vi "Notifications-Events OverSampling x86.vi"() -> ()   [LabVIEW 2020]
uses:
  <userlib>/Beckhoff-LabVIEW-Interface/Utilities/Notification/Buffered User-Event Data.ctl
  <userlib>/Beckhoff-LabVIEW-Interface/_DependsOn/Base/Read/Register E-Notification Buffered.vi
panel:
  out "# elements in queue":i32
  out "Timestamps":i64[](graph)
  out "Signal":dbl[](graph)
  out "Has stopped?":bool
  in  "Stop Event-Loop":bool
  in  "Stop Notification":bool
  in  "Send":bool=TRUE
  in  "Symbol file path":path
  # "Stop Notification before stopping\nEvent-loop"
  # "Note: This example is only an illustration of all possible ways\nhow this Product can be used."
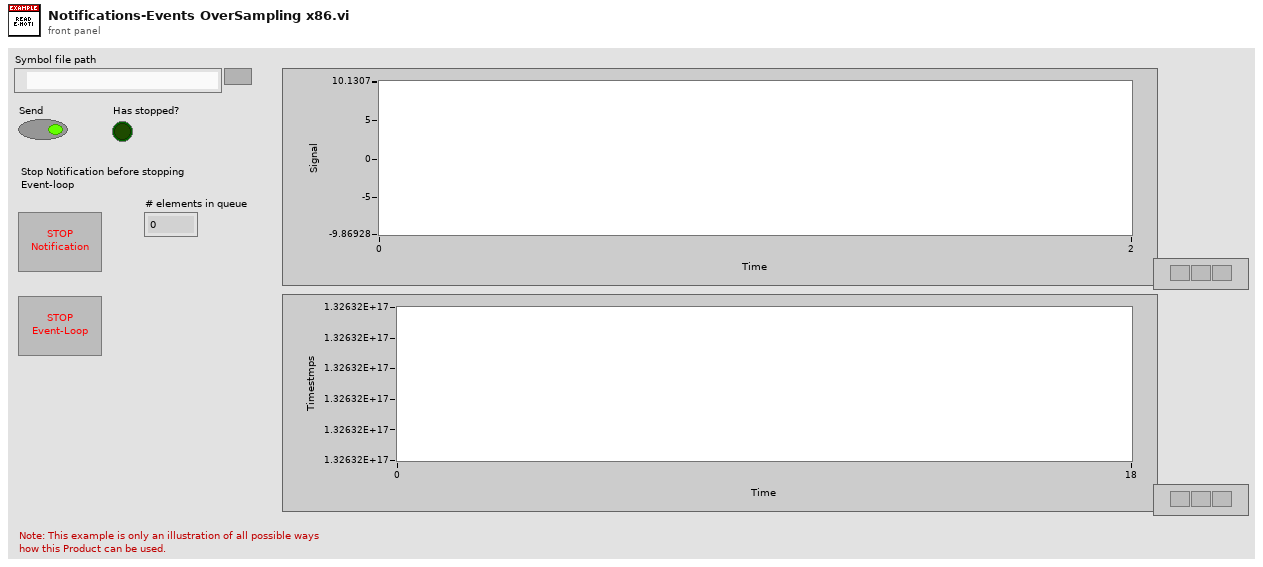
[diagram p1: front panel]
types:
  T1 = typedef "Buffered User-Event Data.ctl" = cluster{"NotiHandle":u32, "Samples":i32, "BufferInfo":cluster{"Previous Overflow Samples":u32, "Missing Samples":u32, "Buffer Usage":dbl}, "RawData":u8[], "Timestamps":i64[]}
  T2 = cluster{"Noti. Data":variant[], "Timestamps":i64[]}
  T3 = cluster{"RDataArray":variant[], "Timestamps":i64[]}
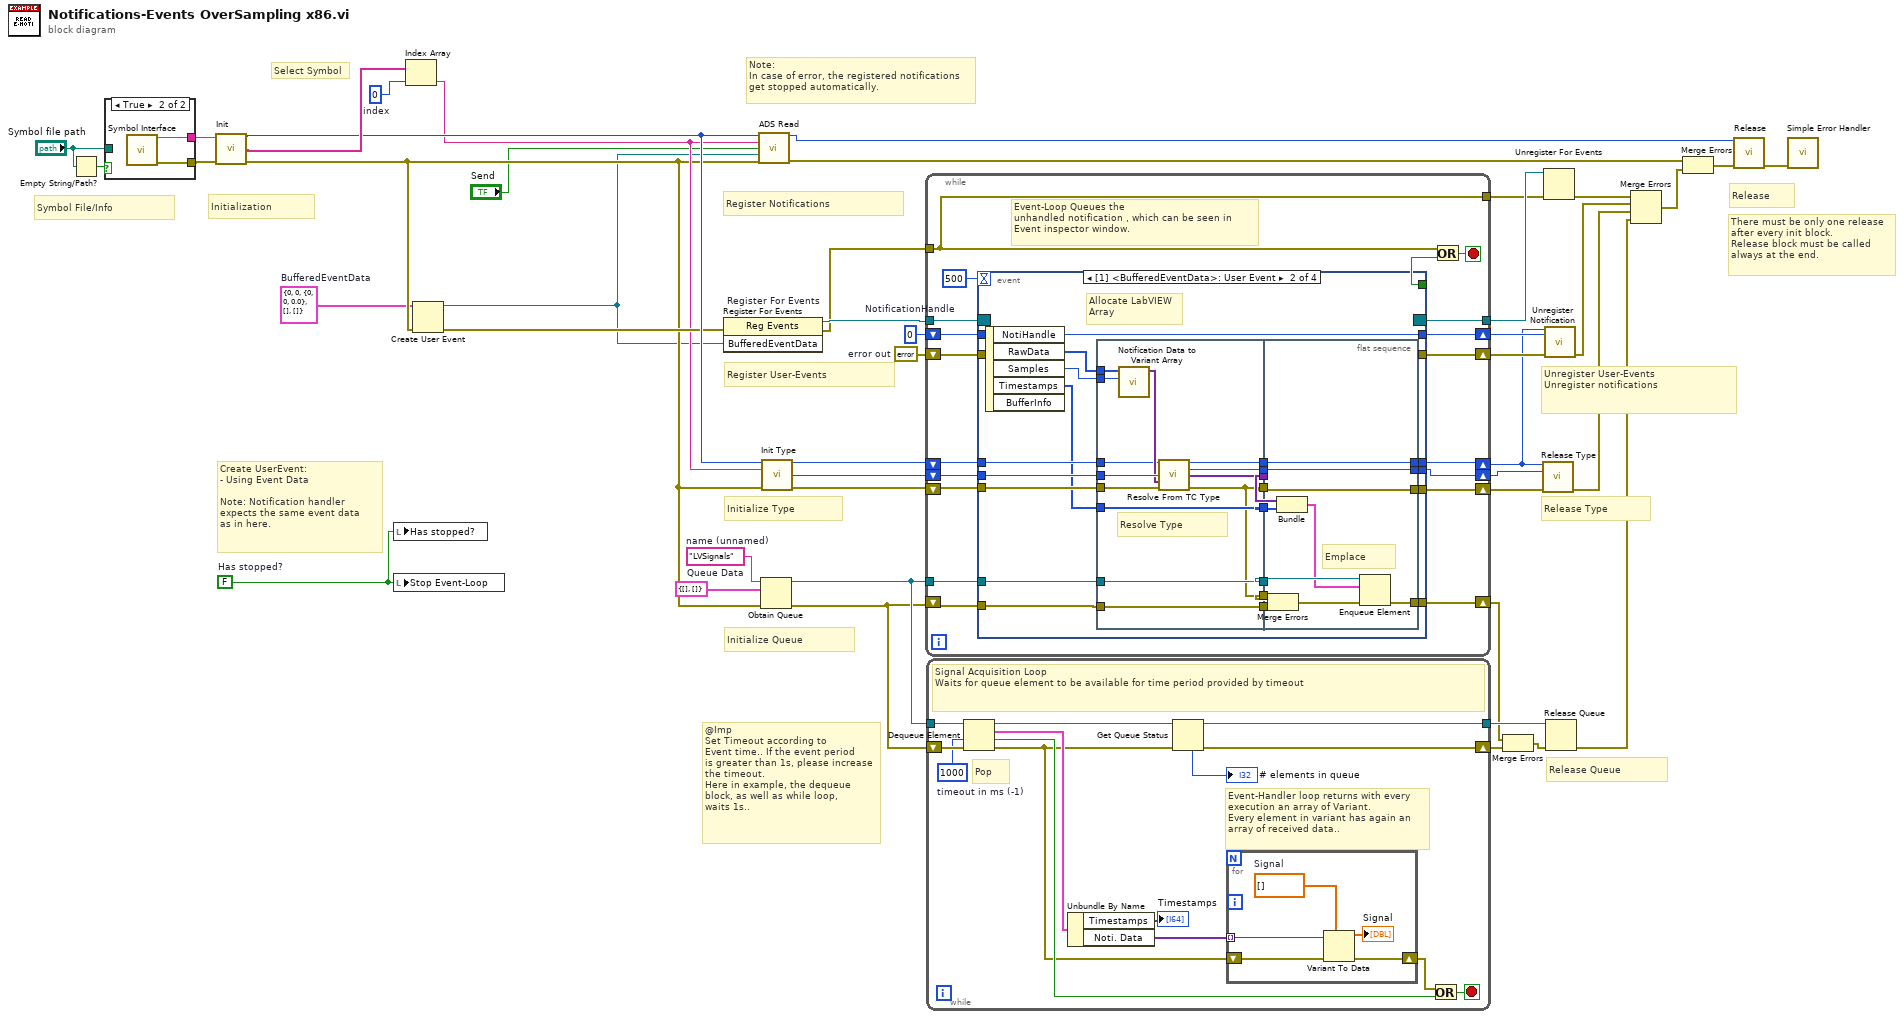
[diagram p0: block diagram]
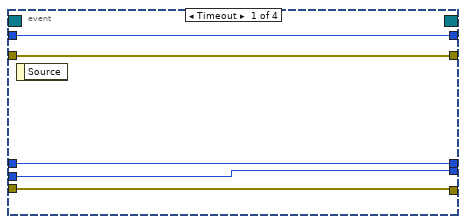
[diagram p2: hidden frame]
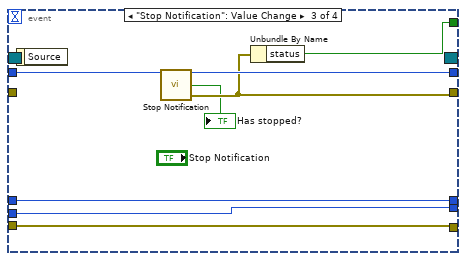
[diagram p3: hidden frame]
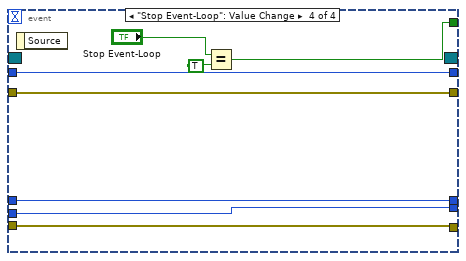
[diagram p4: hidden frame]
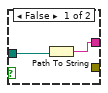
[diagram p5: hidden frame]
diagram:
  w3 = T1 {"NotiHandle"=0, "Samples"=0, "BufferInfo"={"Previous Overflow Samples"=0, "Missing Samples"=0, "Buffer Usage"=0.0}, "RawData"=[], "Timestamps"=[]}  # BufferedEventData
  w13 = "LVSignals"  # name (unnamed)
  w14 = T2 {"Noti. Data"=[], "Timestamps"=[]}  # Queue Data
  w23 = errorcluster {"status"=FALSE, "code"=0, "source"=""}  # error out
  w24 = u32 0  # NotificationHandle
  w36 = 0  # index
  w6 = FALSE  # Has stopped?
  # "@Imp\nSet Timeout according to\nEvent time.. If the event period\nis greater than 1s, please increase\nthe timeout.\nHere in example, the dequeue\nblock, as well as while loop,\nwaits 1s.."
  # "Release Queue"
  # "Initialize Queue"
  # "Release Type"
  # "Initialize Type"
  # "Note:\nIn case of error, the registered notifications\nget stopped automatically."
  # "There must be only one release\nafter every init block.\nRelease block must be called\nalways at the end."
  # "Create UserEvent:\n- Using Event Data\n\nNote: Notification handler\nexpects the same event data\nas in here."
  # "Unregister User-Events\nUnregister notifications"
  # "Register User-Events"
  # "Register Notifications"
  # "Initialization"
  # "Select Symbol"
  # "Release"
  # "Symbol File/Info"
  n1 = Empty String/Path?(string/path="Symbol file path") -> (empty?=w40:bool)
  n2 = case shown="True" w40 {
    tunnel: [_ w49] -> w39
    tunnel: [w47 w48] -> w38
    tunnel: "Symbol file path" -> [w46 _]
    frame False {
      n3 = Path To String(path=w46) -> (string=w47:string)
    }
    frame True {
      n4 = call <userlib>:"Symbol Interface.vi"() -> ("PortInfo"=w48:string, "error out"=w49:errorcluster)  [unwired: 14 in]
    }
  }
  n5 = call <userlib>:"Init.vi"("XMLDescription"=w38, "error in (no error)"=w39) -> ("Handle"=w41:u32, "ReadGrpSymbols"=w45:string[], "error out"=w12:errorcluster)  [unwired: 9 in, 2 out]
  n6 = local write "Has stopped?"(w6) -> ()
  n7 = local write "Stop Event-Loop"(w6) -> ()
  n8 = Index Array "Index Array"(array=w45, index=w36) -> (element=w22:string)
  n9 = Create User Event(user event datatype=w3, error in=w12) -> (user event=w1:refnum<user-event>, error out=w35:errorcluster)
  n10 = register-events "Register For Events"(error in=w35, w1) -> (reference out=w34:refnum<event-registration>, error out=w27:errorcluster)  [unwired: 1 in]
  n11 = call-poly <userlib>:"ADS Read.vi"("Handle"=w41, "SymbolName"=w22, "Start Notifications"="Send", "Noti. E-Buffered Event Ref"=w1, "error in (no error)"=w12) -> ("Handle"=w43:u32, "error out"=w25:errorcluster)  [unwired: 8 in, 1 out]
  n12 = Obtain Queue(name (unnamed)=w13, element data type=w14, error in (no error)=w12) -> (queue out=w11:refnum<queue>, error out=w10:errorcluster)  [unwired: 2 in, 1 out]
  n13 = call <userlib>:"Init Type.vi"("Handle"=w41, "SymbolName"=w22, "error in"=w12) -> ("Handle"=w16:u32, "TypeHdl"=w21:u32, "error IO"=w20:errorcluster)  [unwired: 7 in, 3 out]
  n14 = while {
    tunnel: w34 -> [w68]
    shift-right: [w67] -> w33
    shift-left: w24 -> [w66]
    tunnel: [w64] -> w32
    tunnel: w27 -> [w60]
    tunnel: [w60] -> w26
    shift-right: [w63] -> w31
    shift-left: w23 -> [w59]
    shift-right: [w56] -> w19
    shift-left: w20 -> [w57]
    shift-right: [w55] -> w18
    shift-left: w21 -> [w58]
    shift-right: [w53] -> w15
    shift-left: w16 -> [w54]
    tunnel: w11 -> [w51]
    shift-right: [w50] -> w4
    shift-left: w10 -> [w52]
    stop <- w61 stop-if-true
    # "Event-Loop Queues the \nunhandled notification , which can be seen in \nEvent inspector window."
    n15 = event shown="[1] <BufferedEventData>: User Event" {
      selector: w68 -> [_ _ _ _]
      dyn-events: [_ _ _ _] -> w64
      timeout: 500 -> [_ _ _ _]
      tunnel: [w73 w85 w125 w131] -> w67
      tunnel: w66 -> [w73 _ w126 w131]
      tunnel: [_ _ w123 w132] -> w62
      tunnel: [w72 _ w124 w130] -> w63
      tunnel: w59 -> [w72 _ _ w130]
      tunnel: w58 -> [w70 w94 w120 w128]
      tunnel: w57 -> [w71 w93 w121 w129]
      tunnel: [w71 w80 w121 w129] -> w56
      tunnel: [w70 w89 w120 w128] -> w55
      tunnel: w54 -> [w69 w88 w119 w127]
      tunnel: [w69 w86 w119 w127] -> w53
      tunnel: w52 -> [_ w82 _ _]
      tunnel: w51 -> [_ w76 _ _]
      tunnel: [_ w74 _ _] -> w50
      event Timeout {
        n16 = event-data() -> ()  [unwired: 1 in, 1 out]
      }
      event User Event {
        # "Allocate LabVIEW\nArray"
        n17 = event-data() -> ("NotiHandle"=w85:u32, "RawData"=w84:u8[], "Samples"=w83:i32, "Timestamps"=w79:i64[])  [unwired: 1 in, 1 out]
        n18 = flat-sequence {
          tunnel: w94 -> [w107]
          tunnel: w93 -> [w106]
          tunnel: [w99] -> w92
          tunnel: [w95] -> w91
          tunnel: [w104] -> w90
          tunnel: w88 -> [w103]
          tunnel: [w102] -> w87
          tunnel: w84 -> [w101]
          tunnel: w83 -> [w100]
          tunnel: w82 -> [w98]
          tunnel: [w98] -> w81
          tunnel: w79 -> [w97]
          tunnel: [w97] -> w78
          tunnel: [w96] -> w77
          tunnel: w76 -> [w96]
          tunnel: [w95] -> w75
          tunnel: w92 -> [w113]
          tunnel: w91 -> [w116]
          tunnel: w90 -> [w118]
          tunnel: [w118] -> w89
          tunnel: w87 -> [w117]
          tunnel: [w117] -> w86
          tunnel: w81 -> [w115]
          tunnel: [w109] -> w80
          tunnel: w78 -> [w112]
          tunnel: w77 -> [w111]
          tunnel: w75 -> [w109]
          tunnel: [w108] -> w74
          frame #0 {
            # "Resolve Type"
            n19 = call <userlib>:"Notification Data to Variant Array.vi"("Samples"=w100, "Notification Data"=w101) -> ("Notification Data"=w105:variant[])  [unwired: 9 in]
            n20 = call <userlib>:"Resolve From TC Type.vi"("Handle"=w103, "TypeHdl"=w107, "ADSRData"=w105, "error in"=w106) -> ("Handle"=w102:u32, "TypeHdl"=w104:u32, "RDataArray"=w99:variant[], "error out"=w95:errorcluster)  [unwired: 7 in, 1 out]
          }
          frame #1 {
            # "Emplace"
            n21 = Merge Errors(w116, w115) -> (w114:errorcluster)
            n22 = Bundle("RDataArray"=w113, "Timestamps"=w112) -> (w110:T3)  [unwired: 1 in]
            n23 = Enqueue Element(queue=w111, element=w110, error in (no error)=w114) -> (error out=w108:errorcluster)  [unwired: 1 in, 2 out]
          }
        }
      }
      event "Stop Notification": Value Change {
        n24 = event-data() -> ()  [unwired: 1 in, 1 out]
        n25 = call <userlib>:"Stop Notification.vi"("Reader Handle"=w126) -> ("error out"=w124:errorcluster, "Has stopped?"=→"Has stopped?":bool, "Reader Handle"=w125:u32)  [unwired: 2 in]
        n26 = Unbundle By Name(w124) -> ("status"=w123:bool)
      }
      event "Stop Event-Loop": Value Change {
        n27 = event-data() -> ()  [unwired: 1 in, 1 out]
        n28 = Equal?(x="Stop Event-Loop", y=TRUE) -> (x = y?=w132:bool)
      }
    }
    n29 = Or(x=w60, y=w62) -> (x .or. y?=w61:bool)
  }
  n30 = while {
    shift-right: [w135] -> w8
    shift-left: w10 -> [w146]
    tunnel: w11 -> [w148]
    tunnel: [w138] -> w9
    stop <- w142 stop-if-true
    w139 = 1000  # timeout in ms (-1)
    # "Event-Handler loop returns with every\nexecution an array of Variant.\nEvery element in variant has again an\narray of received data.."
    # "Pop"
    # "Signal Acquisition Loop\nWaits for queue element to be available for time period provided by timeout"
    n31 = Dequeue Element(queue=w148, timeout in ms (-1)=w139, error in (no error)=w146) -> (queue out=w147:refnum<queue>, element=w145:T2, timed out?=w140:bool, error out=w136:errorcluster)
    n32 = Unbundle By Name(w145) -> ("Timestamps"=→"Timestamps":i64[], "Noti. Data"=w144:variant[])
    n33 = Get Queue Status(queue=w147, error in (no error)=w136) -> (queue out=w138:refnum<queue>, error out=w135:errorcluster, # elements in queue=→"# elements in queue":i32)  [unwired: 1 in, 5 out]
    n34 = for {
      tunnel: w144 -> [w153] mode=indexing
      shift-right: [w151] -> w143
      shift-left: w136 -> [w152]
      w150 = dbl[] []  # Signal
      n35 = Variant To Data(error in=w152, type=w150, Variant=w153) -> (data=→"Signal":dbl[], error out=w151:errorcluster)
    }
    n36 = Or(x=w143, y=w140) -> (x .or. y?=w142:bool)
  }
  n37 = Merge Errors "Merge Errors"(w4, w8) -> (w5:errorcluster)
  n38 = call <userlib>:"Release Type.vi"("Handle"=w15, "TypeHandle"=w18, "error in (no error)"=w19) -> ("error out"=w17:errorcluster)  [unwired: 11 in, 1 out]
  n39 = Unregister For Events(event registration refnum=w32, error in=w26) -> (error out=w30:errorcluster)
  n40 = call <userlib>:"Unregister Notification.vi"("Handle"=w15, "Reader Handle"=w33, "error in"=w31) -> ("error out"=w29:errorcluster)  [unwired: 9 in, 3 out]
  n41 = Release Queue(queue=w9, error in (no error)=w5) -> (error out=w7:errorcluster)  [unwired: 1 in, 2 out]
  n42 = Merge Errors "Merge Errors"(w30, w29, w17, w7) -> (w28:errorcluster)
  n43 = Merge Errors "Merge Errors"(w25, w28) -> (w42:errorcluster)
  n44 = call <userlib>:"Release.vi"("Handle"=w43, "error in (no error)"=w42) -> ("error out"=w44:errorcluster)  [unwired: 13 in]
  n45 = call <vilib>:"Simple Error Handler.vi"("error in (no error)"=w44) -> ()  [unwired: 4 in, 5 out]
